vi "createTaskReqstEvent.vi"(8 "error in (no error)":errorcluster, 11 "TaskRef":refnum<vi>) -> (0 "error IO":errorcluster, 2 "pdbm_task_reqst_event":refnum<user-event>, 3 "TaskRef out":refnum<vi>)   [LabVIEW 2015, in "pdbm_task_route.lvlib"]
uses:
  pdbm_task_route.lvlib
  UsrDefine/TaskReqst.ctl
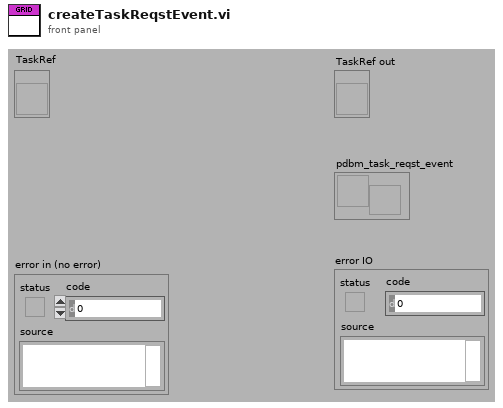
[diagram p1: front panel]
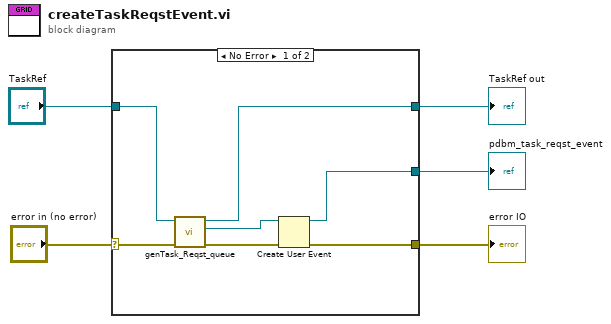
[diagram p0: block diagram]
diagram:
  n1 = case shown="No Error" "error in (no error)" {
    selector: "error in (no error)" -> [w12 w13]
    tunnel: "TaskRef" -> [w11 w14]
    tunnel: [w8 w14] -> w3
    tunnel: [w7 _] -> w2
    tunnel: [w6 w13] -> w1
    frame No Error {
      n2 = call "genTask_Reqst_queue.vi"("error in (no error)"=w12, "TaskRef"=w11) -> ("error IO"=w9:errorcluster, "TaskReqst_queue"=w10:refnum<queue>, "TaskRef out"=w8:refnum<vi>)  [unwired: 7 in]
      n3 = Create User Event(user event datatype=w10, error in=w9) -> (user event=w7:refnum<user-event>, error out=w6:errorcluster)
    }
    frame Error {
    }
  }
  "TaskRef out" <- w3
  "pdbm_task_reqst_event" <- w2
  "error IO" <- w1
